vi "제목없음3.vi"() -> ()   [LabVIEW 2014]
panel:
  in  "Servo Position (0 - 255)":u8(slide)=128 step=1 scale=0.0..255.0
  in  "정지":bool
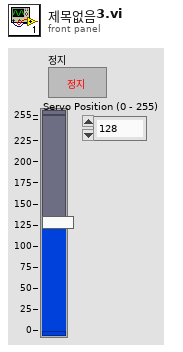
[diagram p1: front panel]
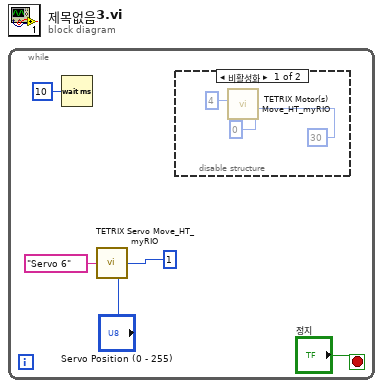
[diagram p0: block diagram]
diagram:
  n1 = while {
    stop <- "정지" stop-if-true
    n2 = Wait (ms)(milliseconds to wait=u32 10 ("대기 시간(ms)")) -> ()  [unwired: 1 out]
    n3 = call <vilib>:"TETRIX Servo Move_HT_myRIO.vi"("Servo Position (0 - 255)"="Servo Position (0 - 255)", "Controller Daisy Chain Position (1 - 4)"=u8 1, "Select Servo"="Servo 6") -> ()  [unwired: 2 in, 1 out]
    n4 = disable-structure shown="비활성화" {
      frame Disabled {
        n5 = call <vilib>:"TETRIX Motor(s) Move_HT_myRIO.vi"("Motor 2 Power (-100 to 100)\n0 = Stop/Brake\n-128 = Stop/Coast"=i8 0 ("Motor 2 Power (-100 to 100)\n0 = Stop/Brake\n-128 = Stop/Coast"), "Motor 1 Power (-100 to 100)\n0 = Stop/Brake\n-128 = Stop/Coast"=i8 30 ("Motor 1 Power (-100 to 100)\n0 = Stop/Brake\n-128 = Stop/Coast"), "Controller Daisy Chain Position: 1 - 4"=u8 4) -> ()  [unwired: 6 in, 1 out]
      }
      frame Enabled {
      }
    }
  }
